vi "Global.vi"() -> ()   [LabVIEW 2017, in "nifxpmath_RectToPolar.xnode"]
uses:
  <vilib>/rvi/FXPMathLib/FxpRectToPolar/XNode/nifxpmath_RectToPolar.xnode
panel:
  in  "TERM PH NAME w/o UNIT":string="phase"
  out "SMALL ICON w/ 4WIRE":picture
  out "SMALL ICON":picture
  out "NORMAL BANNER":picture
  in  "TERM PH NAME":string="phase (pi)"
  in  "TERM MA NAME":string="magnitude"
  in  "TERM Y NAME":string="y"
  in  "TERM X NAME":string="x"
  in  "TERM X ID":string="TERM_X"
  in  "TERM PH ID":string="TERM_PH"
  in  "TERM Y ID":string="TERM_Y"
  in  "TERM MA ID":string="TERM_MA"
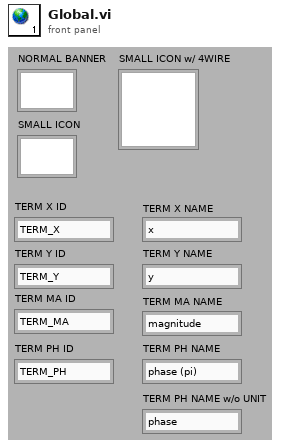
[diagram p1: front panel]
diagram:
